vi "Security_Create.vi"(0 "reference in":refnum<class "Security.lvclass">, 5 "Error In":errorcluster) -> (14 "reference out":refnum<class "Security.lvclass">, 19 "Error Out":errorcluster)   [LabVIEW 2024, in "Security.lvclass"]
uses:
  Security.lvclass
  Security.lvclass/Security.ctl
panel:
  # "Connector Pane"
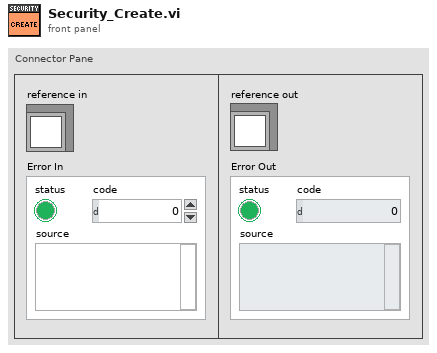
[diagram p1: front panel]
types:
  T1 = typedef "Security.lvclass/ObjectAttributes.ctl" = cluster{"State":bool, "Security Mode":T2}
  T2 = typedef "SecuritySystem.lvclass/Security Mode.ctl" = enum16{"Aggresive", "Defensive", "Balanced"}
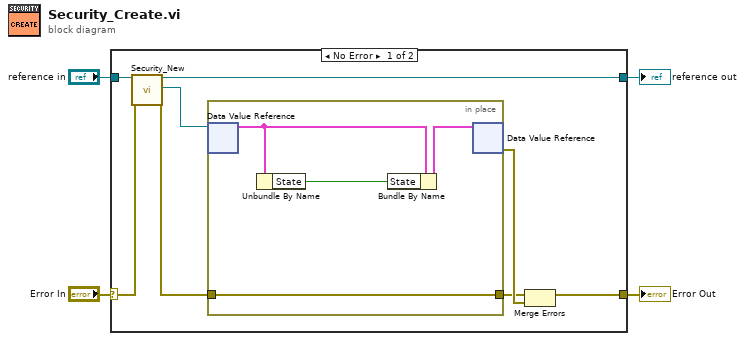
[diagram p0: block diagram]
diagram:
  n1 = case shown="No Error" "Error In" {
    selector: "Error In" -> [w11 w18]
    tunnel: [w8 w18] -> w3
    tunnel: "reference in" -> [w12 w17]
    tunnel: [w10 w17] -> w1
    frame No Error {
      n2 = call "Security_New.vi"("reference in"=w12, "Error In"=w11) -> ("reference out"=w10:refnum<class "Security.lvclass">, "DVRRefOut"=w7:refnum<data-value>, "Error Out"=w6:errorcluster)  [unwired: 14 in, 1 out]
      n3 = in-place {
        in-place-border: w6 -> [w13]
        in-place-border: [w13] -> w5
        n4 = in-place-dvr #1(w7) -> (w15:T1)  [unwired: 1 out]
        n5 = Unbundle By Name(w15) -> ("State"=w14:bool)
        n6 = Bundle By Name(cluster=w15, "State"=w14) -> (w16:T1)
        n7 = in-place-dvr #1(w16) -> (w9:errorcluster)  [unwired: 1 out]
      }
      n8 = Merge Errors(w5, w9) -> (w8:errorcluster)
    }
    frame Error {
      # "VI-TechBaseTemplate_Simple_6x8x6"
    }
  }
  "Error Out" <- w3
  "reference out" <- w1
